vi "frequency_calculator.vi"(7 "Tx Amostragem":dbl=0.0001, 8 "KP slope":dbl, 10 "Min Num of Cycles to Evaluate":i32=5, 11 "All Sensors":dbl[][](array[numeric])) -> (0 "Begin Last Pulse":i32, 2 "Locations":i32[](array[numeric]), 3 "Frequency":dbl, 5 "KeyPhasor Wave":dbl[](graph) caption="Duration")   [LabVIEW 2012]
uses:
  <vilib>/Analysis/NI_AAL_SigProc.lvlib
panel:
  out "Amplitudes":dbl[](array[numeric])
  out "# found":i32
  out "error out":errorcluster
  out "Calculated Freq":dbl
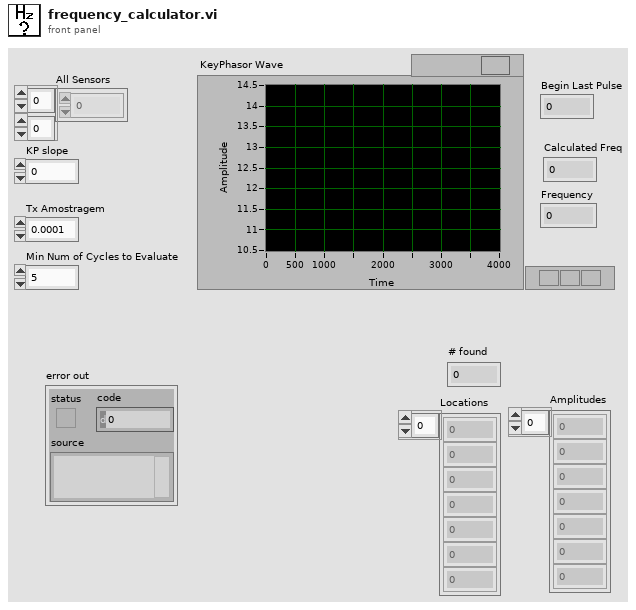
[diagram p1: front panel]
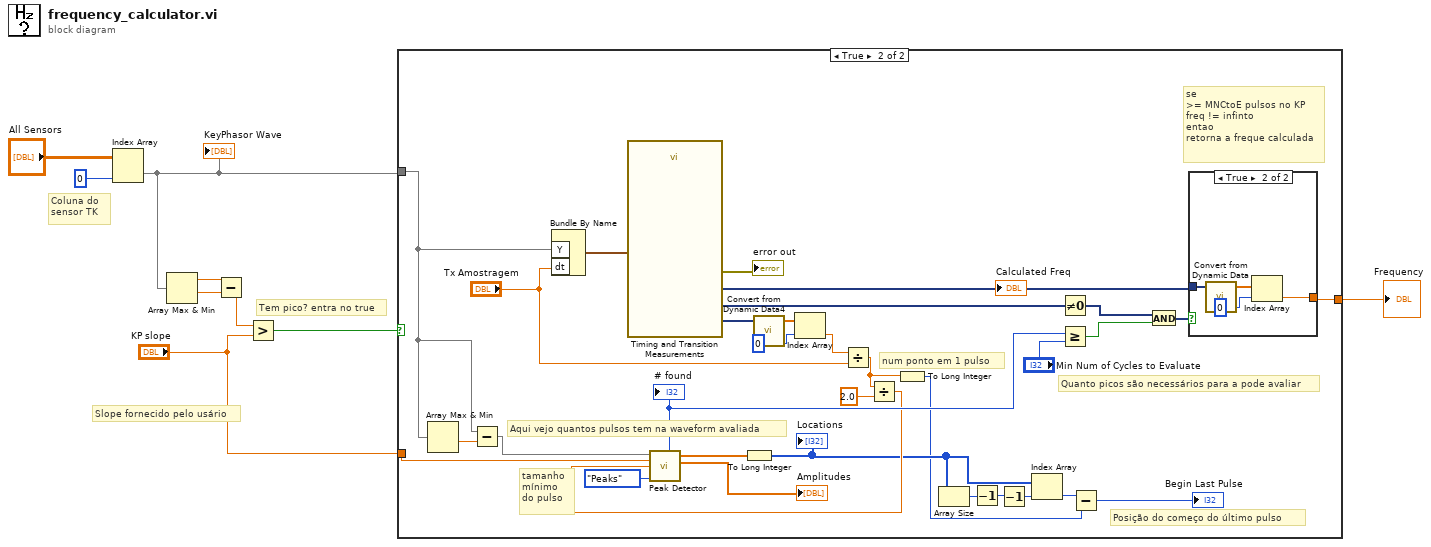
[diagram p0: block diagram]
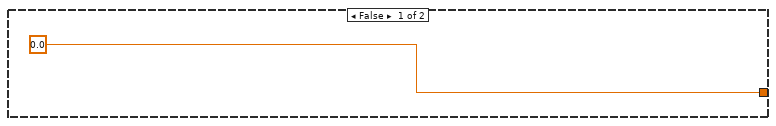
[diagram p2: hidden frame]
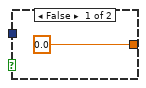
[diagram p3: hidden frame]
diagram:
  # "Slope fornecido pelo usário"
  # "Tem pico? entra no true"
  # "Coluna do \nsensor TK"
  n1 = Index Array(array="All Sensors", index (col)=0 ("disabled index (col)")) -> (element=w5:dbl[])  [unwired: 1 in]
  "KeyPhasor Wave" <- w5
  n2 = Array Max & Min(array=w5) -> (max value=w2:dbl, min value=w7:dbl)  [unwired: 2 out]
  n3 = Subtract(x=w2, y=w7) -> (x-y=w3:dbl)
  n4 = Greater?(x=w3, y="KP slope") -> (0:w4:bool)
  n5 = case shown="True" w4 {
    tunnel: w5 -> [_ w41]
    tunnel: "KP slope" -> [_ w42]
    tunnel: [0.0 w40] -> w1
    frame False {
    }
    frame True {
      # "num ponto em 1 pulso"
      # "tamanho \nmínimo \ndo pulso"
      # "Posição do começo do último pulso"
      # "Quanto picos são necessários para a pode avaliar"
      # "se \n>= MNCtoE pulsos no KP\nfreq != infinto\nentao\nretorna a freque calculada"
      # "Aqui vejo quantos pulsos tem na waveform avaliada"
      n6 = Array Max & Min(array=w41) -> (min value=w35:dbl)  [unwired: 3 out]
      n7 = Subtract(x=w41, y=w35) -> (x-y=w34:dbl[])
      n8 = Bundle By Name("Y"=w41, "dt"="Tx Amostragem") -> (w29:waveform(dbl))  [unwired: 1 in]
      n9 = call "Timing and Transition Measurements"("Signals"=w29) -> ("error out"=→"error out":errorcluster, "Frequency"=w39:dynamicdata, "Period"=w28:dynamicdata, "Duration"=w24:dynamicdata)  [unwired: 7 in]
      "Calculated Freq" <- w39
      n10 = call "Convert from Dynamic Data4"("Dynamic Data Type"=w24) -> ("Array"=w26:dbl[])  [unwired: 3 in]
      n11 = Index Array(array=w26, index=0) -> (element=w19:dbl)
      n12 = Divide(x=w19, y="Tx Amostragem") -> (x/y=w14:dbl)
      n13 = Divide(x=w14, y=2.0) -> (x/y=w21:dbl)
      n14 = call <vilib>:"Peak Detector.vi"("peaks/valleys"=enum32{"Peaks", "Valleys"}."Peaks", "width"=w21, "threshold"=w42, "X"=w34) -> ("Amplitudes"=→"Amplitudes":dbl[], "Locations"=w30:dbl[], "# found"=w32:i32)  [unwired: 3 in, 2 out]
      "# found" <- w32
      n15 = To Long Integer(number=w30) -> (32bit integer=w17:i32[])
      "Locations" <- w17
      n16 = To Long Integer(number=w14) -> (32bit integer=w13:i32)
      n17 = Array Size(array=w17) -> (size(s)=w18:i32)
      n18 = Decrement(x=w18) -> (x-1=w12:i32)
      n19 = Decrement(x=w12) -> (x-1=w11:i32)
      n20 = Index Array(array=w17, index=w11) -> (element=w16:i32)
      n21 = Not Equal To 0?(x=w28) -> (x != 0?=w20:dynamicdata)
      n22 = Greater Or Equal?(x=w32, y="Min Num of Cycles to Evaluate") -> (x >= y?=w33:bool)
      n23 = Subtract(x=w16, y=w13) -> (x-y=→"Begin Last Pulse":i32)
      n24 = And(x=w20, y=w33) -> (x .and. y?=w31:dynamicdata)
      n25 = case shown="True" w31 {
        tunnel: [0.0 ("x") w44] -> w40
        tunnel: w39 -> [_ w45]
        frame False {
        }
        frame True {
          n26 = call "Convert from Dynamic Data"("Dynamic Data Type"=w45) -> ("Array"=w46:dbl[])  [unwired: 3 in]
          n27 = Index Array(array=w46, index=0) -> (element=w44:dbl)
        }
      }
    }
  }
  "Frequency" <- w1
